vi "sandbox.vi"() -> ()   [LabVIEW 2020]
uses:
  Projects/grpc-dynamic-client/src/cpp/out/build/x64-Release/grpc_dynamic_client.dll
panel:
  in  "request":string="{\"resource_name\": \"VST2_01\"}"
  in  "method":string="Init"
  in  "service":string="nirfsa_grpc.NiRFSA"
  in  "target":string="localhost:31763"
  out "response":string
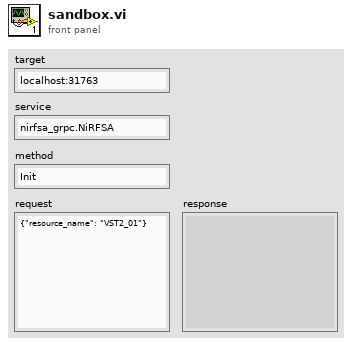
[diagram p1: front panel]
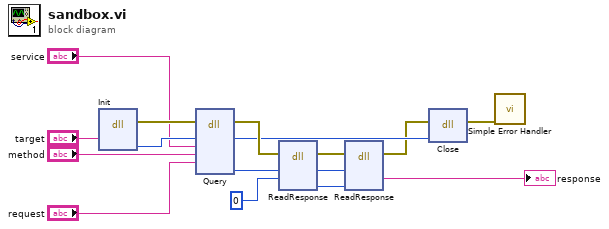
[diagram p0: block diagram]
diagram:
  n1 = dll-call lib="C:/Projects/grpc-dynamic-client/src/cpp/out/build/x64-Release/grpc_dynamic_client.dll" fn="Init"("target"="target") -> (error out=w15:errorcluster, "session_handle"=w14:u64)  [unwired: 6 in, 1 out]
  n2 = dll-call lib="C:/Projects/grpc-dynamic-client/src/cpp/out/build/x64-Release/grpc_dynamic_client.dll" fn="Query"(error in=w15, "session_handle"=w14, "service"="service", "method"="method", "request"="request") -> (error out=w10:errorcluster, "session_handle"=w8:u64, "response_handle"=w9:u64)  [unwired: 7 in, 1 out]
  n3 = dll-call lib="C:/Projects/grpc-dynamic-client/src/cpp/out/build/x64-Release/grpc_dynamic_client.dll" fn="ReadResponse"(error in=w10, "response_handle"=w9, "response"=u64 0) -> (error out=w7:errorcluster, "response_handle"=w4:u64, "size"=w3:u64)  [unwired: 5 in, 1 out]
  n4 = dll-call lib="C:/Projects/grpc-dynamic-client/src/cpp/out/build/x64-Release/grpc_dynamic_client.dll" fn="ReadResponse"(error in=w7, "response_handle"=w4, "size"=w3) -> (error out=w5:errorcluster, "response"=→"response":string)  [unwired: 6 in, 1 out]
  n5 = dll-call lib="C:/Projects/grpc-dynamic-client/src/cpp/out/build/x64-Release/grpc_dynamic_client.dll" fn="Close"(error in=w5, "handle"=w8) -> (error out=w1:errorcluster)  [unwired: 4 in, 1 out]
  n6 = call <vilib>:"Simple Error Handler.vi"("error in (no error)"=w1) -> ()  [unwired: 4 in, 5 out]
